vi "MS-2000 Test Panel.vi"() -> ()   [LabVIEW 2020]
uses:
  <vilib>/Instr/_visa.llb/VISA Configure Serial Port (Instr).vi
panel:
  out "Cmd Success":bool
  out "Connected":bool
  out "Waiting for Reply":bool
  out "Last Error":errorcluster
  out "Command History":string
  out "Reply":string
  in  "Command":string
  in  "Quit":bool
  in  "COM Port":refnum<visa-resource-name>="COM4"
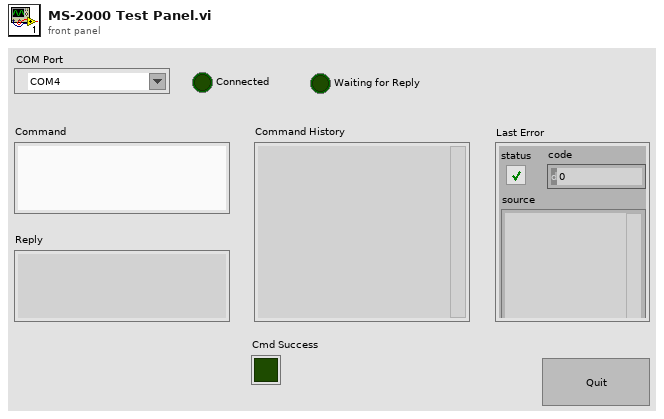
[diagram p1: front panel]
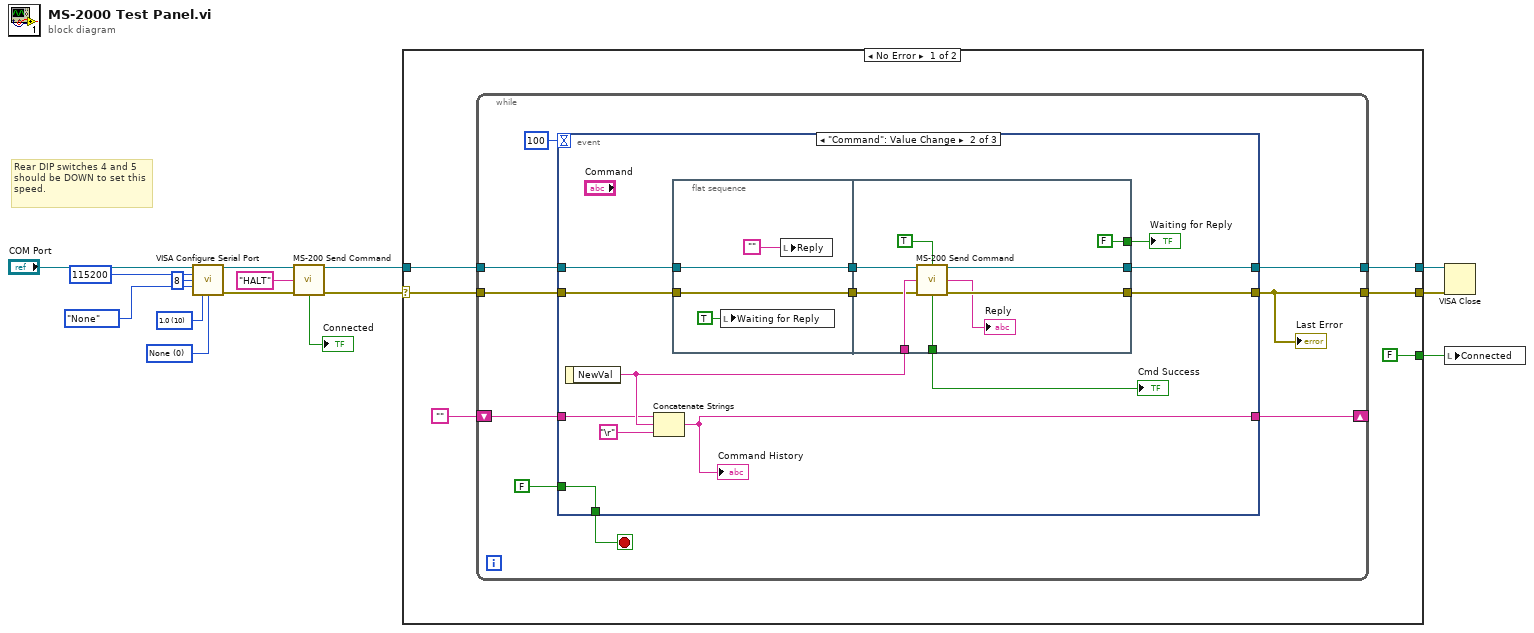
[diagram p0: block diagram]
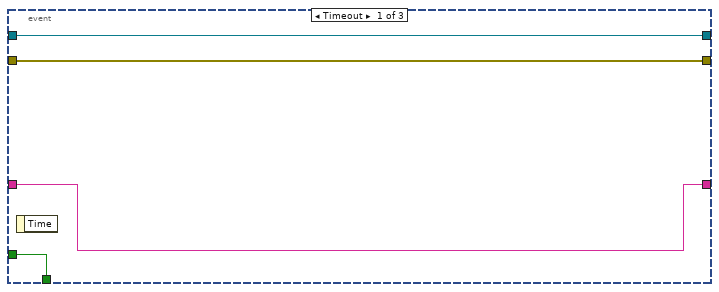
[diagram p2: hidden frame]
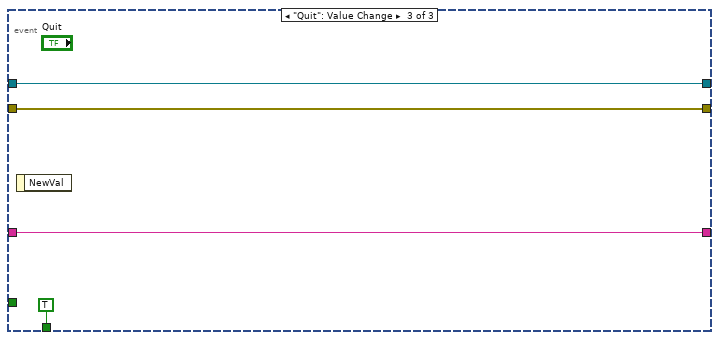
[diagram p3: hidden frame]
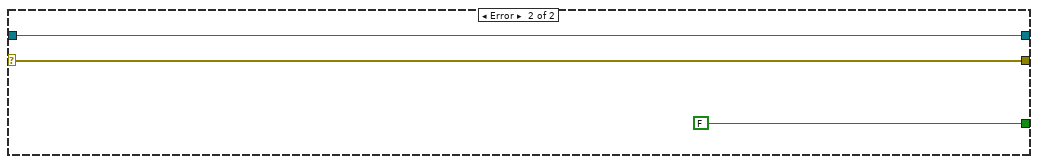
[diagram p4: hidden frame]
diagram:
  w9 = u16 0 items=["None", "XON/XOFF", "RTS/CTS", "XON/XOFF & RTS/CTS", "DTR/DSR", "XON/XOFF & DTR/DSR"] ("flow control (0:none)")
  w12 = u16 10 items=["1.0"=10, "1.5"=15, "2.0"=20] ("stop bits (10: 1 bit)")
  # "Rear DIP switches 4 and 5 should be DOWN to set this speed."
  n1 = call-poly "VISA Configure Serial Port"("VISA resource name"="COM Port", "baud rate (9600)"=u32 115200, "data bits (8)"=u16 8, "parity (0:none)"=enum16{"None", "Odd", "Even", "Mark", "Space"}."None", "stop bits (10: 1 bit)"=w12, "flow control (0:none)"=w9) -> ("VISA resource name out"=w6:refnum<visa-resource-name>, "error out"=w5:errorcluster)  [unwired: 8 in]
  n2 = call "MS-200 Send Command.vi"("VISA Ref"=w6, "Command"="HALT", "Error In"=w5) -> ("VISA Ref Dup"=w3:refnum<visa-resource-name>, "Cmd Success"=→"Connected":bool, "Error Out"=w1:errorcluster)  [unwired: 9 in, 1 out]
  n3 = case shown="No Error" w1 {
    selector: w1 -> [w20 w66]
    tunnel: w3 -> [w21 w67]
    tunnel: [w19 w67] -> w15
    tunnel: [w18 w66] -> w14
    tunnel: [FALSE FALSE] -> w13
    frame No Error {
      n4 = while {
        tunnel: w21 -> [w28]
        tunnel: w20 -> [w27]
        tunnel: [w26] -> w19
        tunnel: [w23] -> w18
        shift-right: [w24] -> _
        shift-left: "" -> [w25]
        stop <- w29 stop-if-true
        n5 = event shown="[1] \"Command\": Value Change" {
          selector: _ -> [_ _ _]
          dyn-events: _ -> [_ _ _]
          timeout: 100 -> [_ _ _]
          tunnel: FALSE -> [w34 w47 _]
          tunnel: [w34 w47 TRUE] -> w29
          tunnel: w28 -> [w32 w46 w64]
          tunnel: w27 -> [w31 w45 w63]
          tunnel: [w32 w41 w64] -> w26
          tunnel: [w31 w42 w63] -> w23
          tunnel: w25 -> [w33 w38 w61]
          tunnel: [w33 w37 w61] -> w24
          event Timeout {
            n6 = event-data() -> ()  [unwired: 1 in, 1 out]
          }
          event "Command": Value Change {
            n7 = event-data() -> ("NewVal"=w40:string)  [unwired: 1 in]
            n8 = Concatenate Strings(w38, w40, "\r") -> (w37:string)
            "Command History" <- w37
            n9 = flat-sequence {
              tunnel: w45 -> [w50]
              tunnel: w46 -> [w51]
              tunnel: [w51] -> w44
              tunnel: [w50] -> w43
              tunnel: w40 -> [w59]
              tunnel: w44 -> [w60]
              tunnel: w43 -> [w58]
              tunnel: [w57] -> w42
              tunnel: [w56] -> w41
              tunnel: [FALSE] -> w36
              tunnel: [w53] -> w35
              frame #0 {
                n10 = local write "Waiting for Reply"(TRUE ("Waiting for Cmd")) -> ()
                n11 = local write "Reply"("") -> ()
              }
              frame #1 {
                n12 = call "MS-200 Send Command.vi"("VISA Ref"=w60, "Wait for Reply (T)"=TRUE, "Command"=w59, "Error In"=w58) -> ("VISA Ref Dup"=w56:refnum<visa-resource-name>, "Reply"=→"Reply":string, "Cmd Success"=w53:bool, "Error Out"=w57:errorcluster)  [unwired: 8 in]
              }
            }
            "Waiting for Reply" <- w36
            "Cmd Success" <- w35
          }
          event "Quit": Value Change {
            n13 = event-data() -> ()  [unwired: 1 in, 1 out]
          }
        }
        "Last Error" <- w23
      }
    }
    frame Error {
    }
  }
  n14 = VISA Close(VISA resource name=w15, error in (no error)=w14) -> ()  [unwired: 1 out]
  n15 = local write "Connected"(w13) -> ()
